vi "Hand Dryer.vi"() -> ()   [LabVIEW 2013]
panel:
  in  "Set Temperature Limit":dbl min=0.0 max=100.0
  out "Thermistor Reading":dbl
  in  "Temperature\nControl":dbl(slide) scale=0.0..100.0
  in  "?":bool
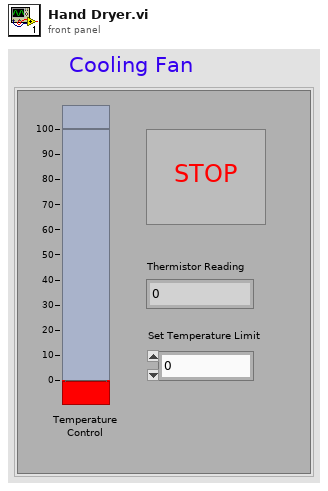
[diagram p1: front panel]
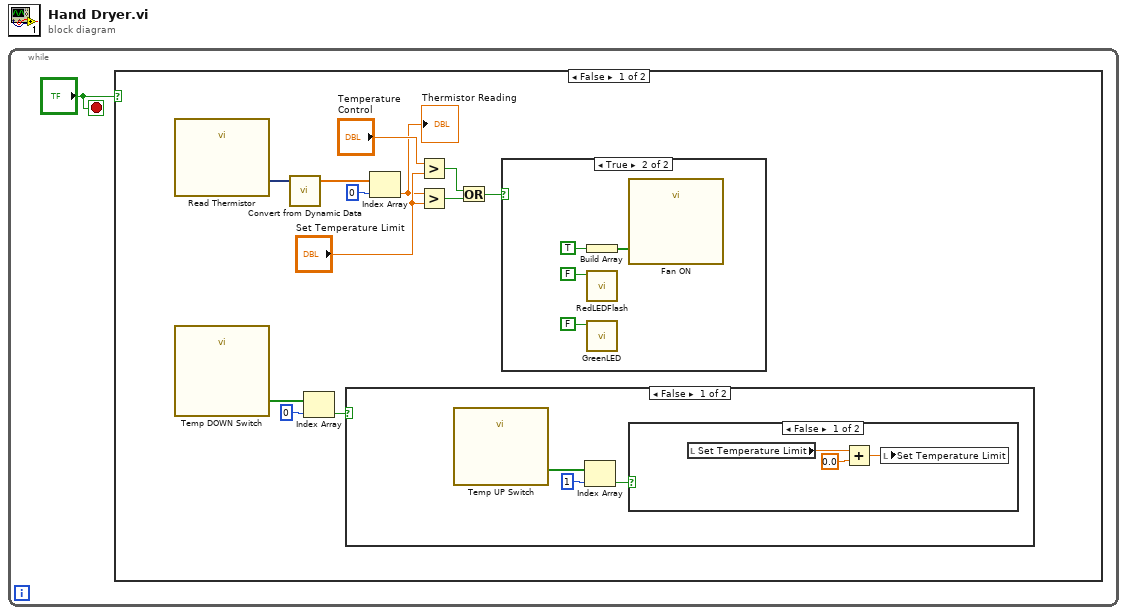
[diagram p0: block diagram]
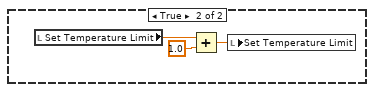
[diagram p2: hidden frame]
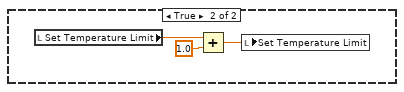
[diagram p3: hidden frame]
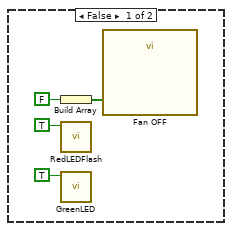
[diagram p4: hidden frame]
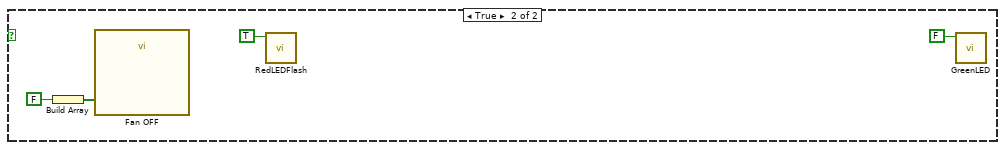
[diagram p5: hidden frame]
diagram:
  n1 = while {
    stop <- "?" stop-if-true
    n2 = case shown="False" "?" {
      frame False {
        n3 = call "Read Thermistor"() -> ("data"=w10:dynamicdata)  [unwired: 17 in, 2 out]
        n4 = call "Temp DOWN Switch"() -> ("data"=w4:bool[])  [unwired: 17 in, 2 out]
        n5 = call "Convert from Dynamic Data"("Dynamic Data Type"=w10) -> ("Array"=w9:dbl[])  [unwired: 3 in]
        n6 = Index Array(array=w4, index=0) -> (element=w2:bool)
        n7 = case shown="False" w2 {
          frame False {
            n8 = call "Temp UP Switch"() -> ("data"=w16:bool[])  [unwired: 17 in, 2 out]
            n9 = Index Array(array=w16, index=1) -> (element=w14:bool)
            n10 = case shown="False" w14 {
              frame False {
                n11 = local read "Set Temperature Limit"() -> (w18:dbl)
                n12 = Add(x=w18, y=0.0) -> (x+y=w17:dbl)
                n13 = local write "Set Temperature Limit"(w17) -> ()
              }
              frame True {
                n14 = local read "Set Temperature Limit"() -> (w21:dbl)
                n15 = Add(x=w21, y=1.0) -> (x+y=w20:dbl)
                n16 = local write "Set Temperature Limit"(w20) -> ()
              }
            }
          }
          frame True {
            n17 = local read "Set Temperature Limit"() -> (w23:dbl)
            n18 = Add(x=w23, y=1.0) -> (x+y=w24:dbl)
            n19 = local write "Set Temperature Limit"(w24) -> ()
          }
        }
        n20 = Index Array(array=w9, index=0) -> (element=w6:dbl)
        "Thermistor Reading" <- w6
        n21 = Greater?(x="Temperature\nControl", y="Set Temperature Limit") -> (0:w11:bool)
        n22 = Greater?(x=w6, y="Set Temperature Limit") -> (0:w5:bool)
        n23 = Or(x=w11, y=w5) -> (x .or. y?=w13:bool)
        n24 = case shown="True" w13 {
          frame False {
            n25 = Build Array(FALSE) -> (w28:bool[])
            n26 = call "RedLEDFlash.vi"("Boolean"=TRUE) -> ()  [unwired: 11 in]
            n27 = call "GreenLED.vi"("Boolean"=TRUE) -> ()  [unwired: 11 in]
            n28 = call "Fan OFF"("data"=w28) -> ()  [unwired: 17 in, 2 out]
          }
          frame True {
            n29 = Build Array(TRUE) -> (w32:bool[])
            n30 = call "RedLEDFlash.vi"("Boolean"=FALSE) -> ()  [unwired: 11 in]
            n31 = call "GreenLED.vi"("Boolean"=FALSE) -> ()  [unwired: 11 in]
            n32 = call "Fan ON"("data"=w32) -> ()  [unwired: 17 in, 2 out]
          }
        }
      }
      frame True {
        n33 = Build Array(FALSE) -> (w36:bool[])
        n34 = call "Fan OFF"("data"=w36) -> ()  [unwired: 17 in, 2 out]
        n35 = call "RedLEDFlash.vi"("Boolean"=TRUE) -> ()  [unwired: 11 in]
        n36 = call "GreenLED.vi"("Boolean"=FALSE) -> ()  [unwired: 11 in]
      }
    }
  }
